vi "Builder.Send Response.vi"(8 "error in (no error)":errorcluster, 10 "response":T1, 11 "Builder in":refnum<class "Builder.lvclass">) -> (0 "error out":errorcluster, 3 "Builder out":refnum<class "Builder.lvclass">)   [LabVIEW 2016, in "DSF.Engine.lvlib" / "Builder.lvclass"]
uses:
  Builder.lvclass
  Interface/DSF.Engine.Interface.Builder.Response Data.ctl
  Interface/DSF.Engine.Interface.Builder.Response.ctl
  Builder.lvclass/Builder.ctl
  Interface/DSF.Engine.Interface.Builder.Write.Response.vi
  Interface/DSF.Engine.Interface.Builder.lvclass
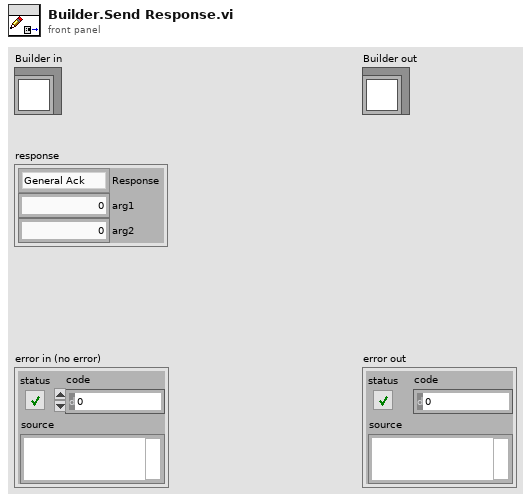
[diagram p1: front panel]
types:
  T1 = typedef "DSF.Engine.lvlib/DSF.Engine.Interface.Builder.lvclass/DSF.Engine.Interface.Builder.Response Data.ctl" = cluster{"Response":T2, "arg1":u64, "arg2":u64}
  T2 = typedef "DSF.Engine.lvlib/DSF.Engine.Interface.Builder.lvclass/DSF.Engine.Interface.Builder.Response.ctl" = enum8{"General Ack", "Initialize Complete", "Parse Complete", "Build Complete", "Shutdown Ack"}
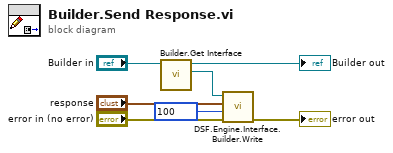
[diagram p0: block diagram]
diagram:
  n1 = call "Builder.Get Interface.vi"("Builder in"="Builder in") -> ("Builder Interface"=w5:refnum<class "DSF.Engine.Interface.Builder.lvclass">, "Builder out"=→"Builder out":refnum<class "Builder.lvclass">)  [unwired: 9 in]
  n2 = call-poly "DSF.Engine.Interface.Builder.Write.vi"("error in (no error)"="error in (no error)", "timeout in ms (0)"=100, "response"="response", "Builder Interface in"=w5) -> ("error out"=→"error out":errorcluster)  [unwired: 5 in, 2 out]
